vi "HAL.vi"   [LabVIEW 2016]
uses:
  PLC/PLC.lvlib
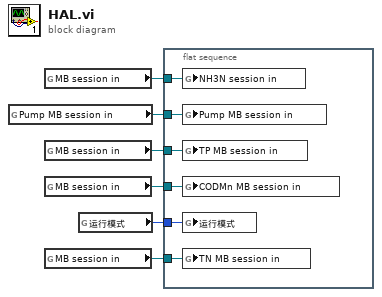
[diagram p0: block diagram]
diagram:
  n1 = global read "采配水全局变量.vi" "Pump MB session in"() -> (w5:refnum<class "MB_Master.lvclass">)
  n2 = global read "VAR氨氮全局变量.vi" "MB session in"() -> (w4:refnum<class "MB_Master.lvclass">)
  n3 = global read "VAR总磷全局变量.vi" "MB session in"() -> (w3:refnum<class "MB_Master.lvclass">)
  n4 = global read "VARCODMn全局变量.vi" "MB session in"() -> (w1:refnum<class "MB_Master.lvclass">)
  n5 = global read "VAR总氮全局变量.vi" "MB session in"() -> (w2:refnum<class "MB_Master.lvclass">)
  n6 = global read "系统设置全局变量.vi" "运行模式"() -> (w6:enum16{"维护模式", "常规模式", "应急模式", "质控模式"})
  n7 = flat-sequence {
    tunnel: w6 -> [w12]
    tunnel: w5 -> [w10]
    tunnel: w4 -> [w11]
    tunnel: w3 -> [w9]
    tunnel: w2 -> [w8]
    tunnel: w1 -> [w7]
    frame #0 {
      n8 = global write "系统交互.vi" "NH3N session in"(w11) -> ()
      n9 = global write "系统交互.vi" "Pump MB session in"(w10) -> ()
      n10 = global write "系统交互.vi" "TP MB session in"(w9) -> ()
      n11 = global write "系统交互.vi" "CODMn MB session in"(w7) -> ()
      n12 = global write "系统交互.vi" "运行模式"(w12) -> ()
      n13 = global write "系统交互.vi" "TN MB session in"(w8) -> ()
    }
  }
